vi "Find Tests.vi"(8 "error in (no error)":errorcluster, 10 "Project or Class Path":path, 11 "Execution UI In":refnum<class "Execution UI.lvclass">) -> (0 "error out":errorcluster, 3 "Execution UI Out":refnum<class "Execution UI.lvclass">)   [LabVIEW 2020, in "Execution UI.lvclass"]
uses:
  Execution UI.lvclass
  Execution UI.lvclass/Execution UI.ctl
  Helper Classes/Test Finder/Test Finder.lvclass
  Rewrite Project/Utilities/LUnit Utilities.lvlib
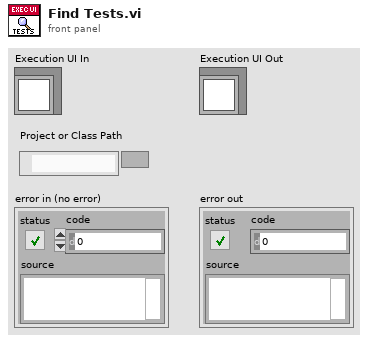
[diagram p1: front panel]
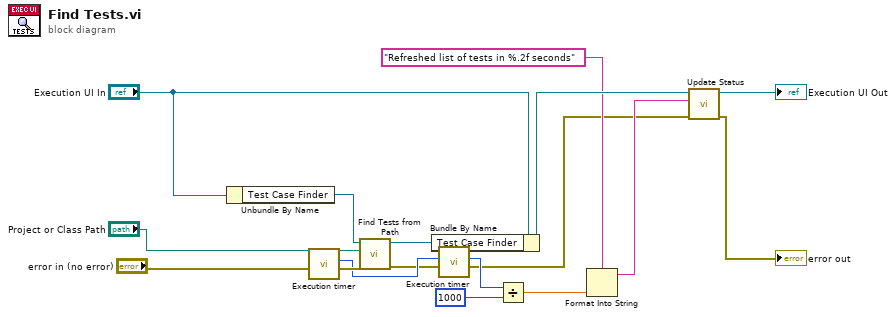
[diagram p0: block diagram]
diagram:
  n1 = Unbundle By Name("Execution UI In") -> ("Test Case Finder"=w2:refnum<class "Test Finder.lvclass">)
  n2 = call "Execution timer.vi"("error in (no error)"="error in (no error)") -> ("error out"=w14:errorcluster, "Current or Duration [ms]"=w13:u32)  [unwired: 9 in]
  n3 = call-dynamic "Find Tests from Path.vi"("error in (no error)"=w14, "Project or Class Path"="Project or Class Path", "Test Case Finder In"=w2) -> ("error out"=w5:errorcluster, "Test Case Finder Out"=w6:refnum<class "Test Finder.lvclass">)  [unwired: 7 in]
  n4 = Bundle By Name(cluster="Execution UI In", "Test Case Finder"=w6) -> (w17:refnum<class "Execution UI.lvclass">)
  n5 = call "Execution timer.vi"("error in (no error)"=w5, "millisecond timer value"=w13) -> ("error out"=w7:errorcluster, "Current or Duration [ms]"=w11:u32)  [unwired: 8 in]
  n6 = Divide(x=w11, y=u32 1000) -> (x/y=w12:dbl)
  n7 = Format Into String(format string="Refreshed list of tests in %.2f seconds" ("Status"), w12) -> (resulting string=w8:string)  [unwired: 2 in, 1 out]
  n8 = call "Update Status.vi"("error in (no error)"=w7, "Status"=w8, "Execution UI In"=w17) -> ("error out"=→"error out":errorcluster, "Execution UI Out"=→"Execution UI Out":refnum<class "Execution UI.lvclass">)  [unwired: 7 in]
